vi "Get acquisition start numbers.vi"(10 "Acquisition order":T1(ring)) -> (0 "Bookmark start number":i32, 1 "Z-step start number":i32, 2 "Time start number":i32, 3 "Channel start number":i32)   [LabVIEW 2017]
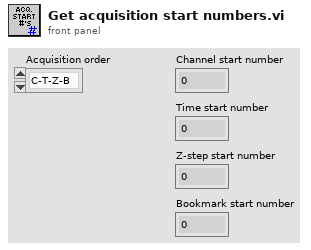
[diagram p1: front panel]
types:
  T1 = enum16{"C-T-Z-B", "C-T-B-Z", "C-Z-T-B", "C-Z-B-T", "C-B-T-Z", "C-B-Z-T", "T-C-Z-B", "T-C-B-Z", "T-Z-C-B", "T-Z-B-C", "T-B-C-Z", "T-B-Z-C", "Z-C-T-B", "Z-C-B-T", "Z-T-C-B", "Z-T-B-C", "Z-B-C-T", "Z-B-T-C", "B-C-T-Z", "B-C-Z-T", "B-Z-C-T", "B-Z-T-C", "B-T-C-Z", "B-T-Z-C"}
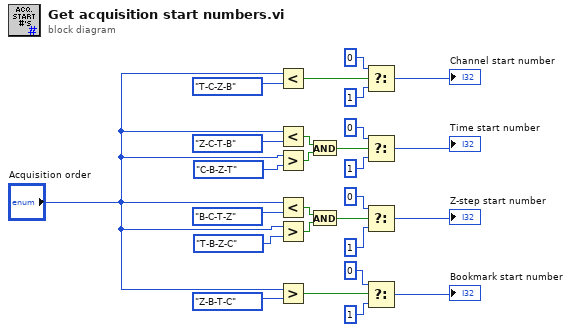
[diagram p0: block diagram]
diagram:
  n1 = Less?(x="Acquisition order", y=T1."T-C-Z-B") -> (x < y?=w25:bool)
  n2 = Less?(x="Acquisition order", y=T1."Z-C-T-B") -> (x < y?=w20:bool)
  n3 = Greater?(x="Acquisition order", y=T1."C-B-Z-T") -> (0:w21:bool)
  n4 = Less?(x="Acquisition order", y=T1."B-C-T-Z") -> (x < y?=w7:bool)
  n5 = Greater?(x="Acquisition order", y=T1."T-B-Z-C") -> (0:w6:bool)
  n6 = Greater?(x="Acquisition order", y=T1."Z-B-T-C") -> (0:w14:bool)
  n7 = And(x=w20, y=w21) -> (x .and. y?=w22:bool)
  n8 = And(x=w7, y=w6) -> (x .and. y?=w5:bool)
  n9 = Select(t=0, s=w25, f=1) -> (s? t:f=→"Channel start number":i32)
  n10 = Select(t=0, s=w22, f=1) -> (s? t:f=→"Time start number":i32)
  n11 = Select(t=0, s=w5, f=1) -> (s? t:f=→"Z-step start number":i32)
  n12 = Select(t=0, s=w14, f=1) -> (s? t:f=→"Bookmark start number":i32)
